vi "Examan.vi"() -> ()   [LabVIEW 2017]
panel:
  in  "S":bool
  out "D":bool
  out "M":bool
  out "L":string
  in  "P1":bool
  in  "P0":bool
  in  "B":bool
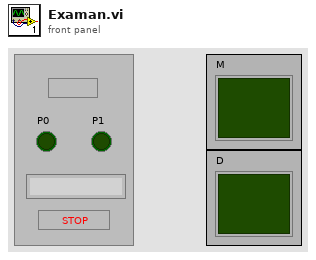
[diagram p1: front panel]
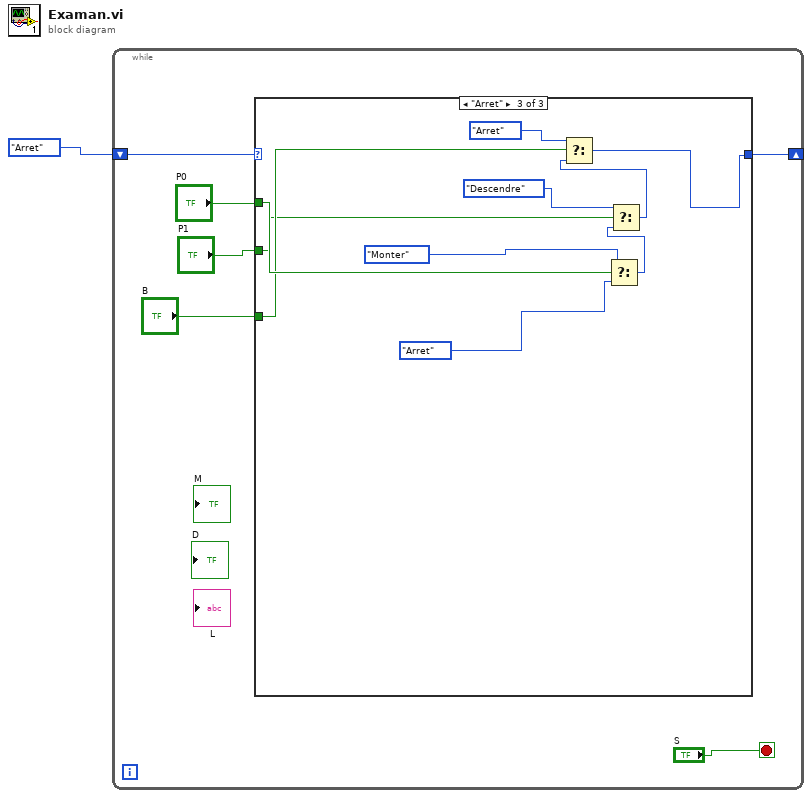
[diagram p0: block diagram]
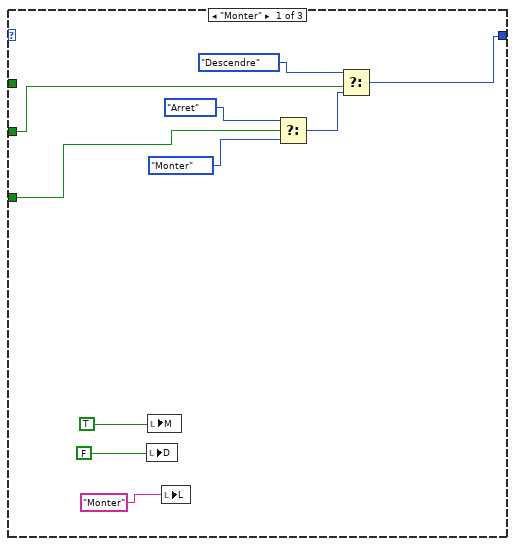
[diagram p2: hidden frame]
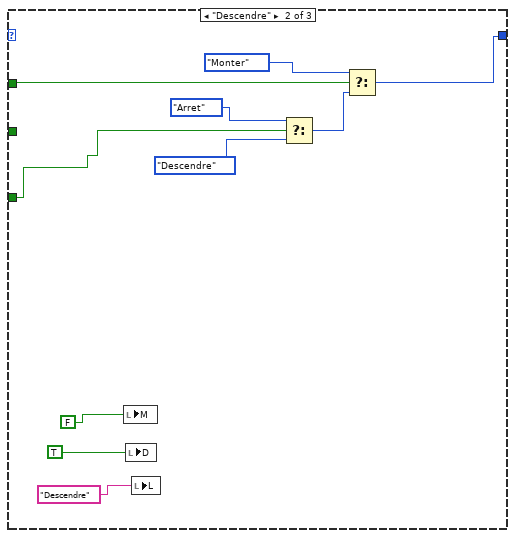
[diagram p3: hidden frame]
diagram:
  n1 = while {
    shift-right: [w6] -> _
    shift-left: enum16{"Monter", "Descendre", "Arret"}."Arret" -> [w7]
    stop <- "S" stop-if-true
    n2 = case shown="\"Arret\"" w7 {
      tunnel: [w10 w23 w33] -> w6
      tunnel: "P0" -> [_ w18 w36]
      tunnel: "B" -> [w9 w19 w35]
      tunnel: "P1" -> [w8 _ w29]
      frame "Monter" {
        n3 = local write "D"(FALSE) -> ()
        n4 = local write "M"(TRUE) -> ()
        n5 = local write "L"("Monter") -> ()
        n6 = Select(t=enum16{"Monter", "Descendre", "Arret"}."Arret", s=w9, f=enum16{"Monter", "Descendre", "Arret"}."Monter") -> (s? t:f=w13:enum16{"Monter", "Descendre", "Arret"})
        n7 = Select(t=enum16{"Monter", "Descendre", "Arret"}."Descendre", s=w8, f=w13) -> (s? t:f=w10:enum16{"Monter", "Descendre", "Arret"})
      }
      frame "Descendre" {
        n8 = local write "M"(FALSE) -> ()
        n9 = local write "D"(TRUE) -> ()
        n10 = local write "L"("Descendre") -> ()
        n11 = Select(t=enum16{"Monter", "Descendre", "Arret"}."Arret", s=w19, f=enum16{"Monter", "Descendre", "Arret"}."Descendre") -> (s? t:f=w26:enum16{"Monter", "Descendre", "Arret"})
        n12 = Select(t=enum16{"Monter", "Descendre", "Arret"}."Monter", s=w18, f=w26) -> (s? t:f=w23:enum16{"Monter", "Descendre", "Arret"})
      }
      frame "Arret" {
        n13 = Select(t=enum16{"Monter", "Descendre", "Arret"}."Monter", s=w36, f=enum16{"Monter", "Descendre", "Arret"}."Arret") -> (s? t:f=w31:enum16{"Monter", "Descendre", "Arret"})
        n14 = Select(t=enum16{"Monter", "Descendre", "Arret"}."Descendre", s=w29, f=w31) -> (s? t:f=w28:enum16{"Monter", "Descendre", "Arret"})
        n15 = Select(t=enum16{"Monter", "Descendre", "Arret"}."Arret", s=w35, f=w28) -> (s? t:f=w33:enum16{"Monter", "Descendre", "Arret"})
      }
    }
  }
